vi "MW区收.vi"(6 "数值类型":enum16{"长整型", "双精度"}(ring), 7 "MD模式":enum16{"读MD", "写MD"}(ring), 9 "16#字符串":string, 10 "寄存器MD地址":i32=10, 11 "处理识别码":i32) -> (1 "数值":sgl, 2 "数值":u32, 3 "读写OK":bool)   [LabVIEW 2016]
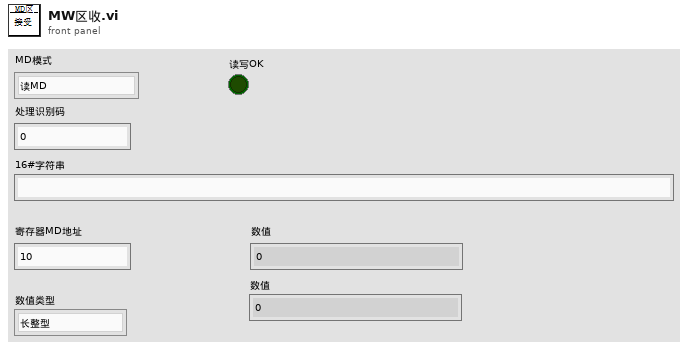
[diagram p1: front panel]
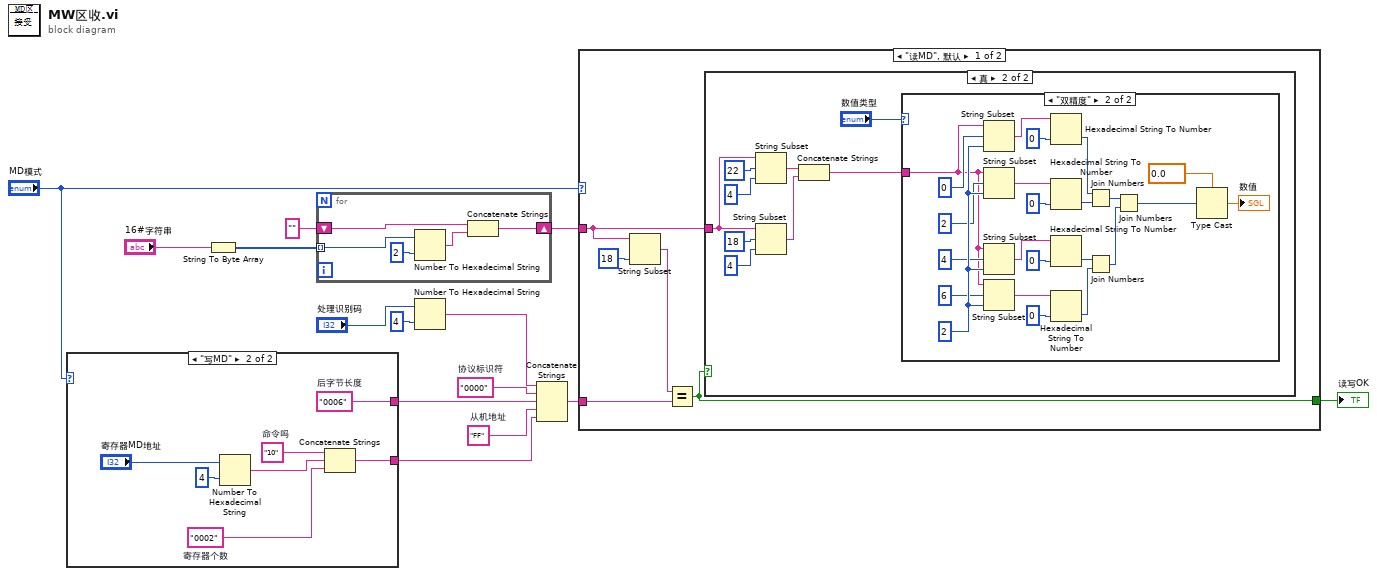
[diagram p0: block diagram]
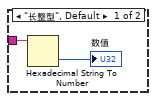
[diagram p3: hidden frame]
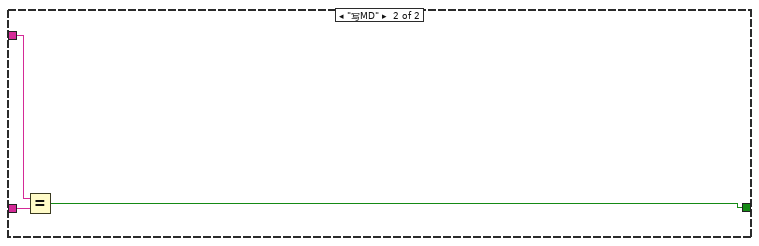
[diagram p4: hidden frame]
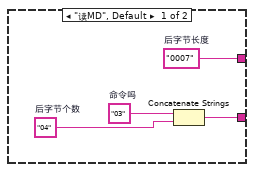
[diagram p5: hidden frame]
diagram:
  w10 = "FF"  # 从机地址
  w11 = "0000"  # 协议标识符
  n1 = case shown="\"写MD\"" "MD模式" {
    tunnel: [w18 w25] -> w9
    tunnel: [w15 w20] -> w4
    frame "读MD", Default {
      w17 = "03"  # 命令吗
      w16 = "04"  # 后字节个数
      w18 = "0007"  # 后字节长度
      n2 = Concatenate Strings(w17, w16) -> (w15:string)
    }
    frame "写MD" {
      w23 = "10"  # 命令吗
      w21 = "0002"  # 寄存器个数
      w25 = "0006"  # 后字节长度
      n3 = Number To Hexadecimal String(1:i16 4 ("宽度(-)"), 2:"寄存器MD地址") -> (0:w22:string)
      n4 = Concatenate Strings(w23, w22, w21) -> (w20:string)
    }
  }
  n5 = String To Byte Array(string="16#字符串") -> (unsigned byte array=w8:u8[])
  n6 = for {
    tunnel: w8 -> [w30] mode=indexing
    shift-right: [w28] -> w5
    shift-left: "" -> [w29]
    n7 = Number To Hexadecimal String ("数值至十六进制字符串转换")(1:i16 2 ("宽度(-)"), 2:w30) -> (0:w26:string)
    n8 = Concatenate Strings(w29, w26) -> (w28:string)
  }
  n9 = Number To Hexadecimal String(1:i16 4 ("宽度(-)"), 2:"处理识别码") -> (0:w12:string)
  n10 = Concatenate Strings(w12, w11, w9, w10, w4) -> (w2:string)
  n11 = case shown="\"读MD\", 默认" "MD模式" {
    tunnel: w5 -> [w31 w72]
    tunnel: w2 -> [w33 w71]
    tunnel: [w32 w70] -> w1
    frame "读MD", Default {
      n12 = String Subset(string=w31, length (rest)=18 ("长度（剩余）")) -> (substring=w34:string)  [unwired: 1 in]
      n13 = Equal?(x=w34, y=w33) -> (x = y?=w32:bool)
      n14 = case shown="真" w32 {
        tunnel: w31 -> [_ w38]
        frame False {
        }
        frame True {
          n15 = String Subset(string=w38, offset (0)=22 ("偏移量(0)"), length (rest)=4 ("长度（剩余）")) -> (substring=w40:string)
          n16 = String Subset(string=w38, offset (0)=18 ("偏移量(0)"), length (rest)=4 ("长度（剩余）")) -> (substring=w39:string)
          n17 = Concatenate Strings(w40, w39) -> (w36:string)
          n18 = case shown="\"双精度\"" "数值类型" {
            tunnel: w36 -> [w45 w47]
            frame "长整型", Default {
              n19 = Hexadecimal String To Number(string=w45) -> (number=→"数值":u32)  [unwired: 2 in, 1 out]
            }
            frame "双精度" {
              w52 = 2 ("长度（剩余）")
              n20 = String Subset(string=w47, offset (0)=0 ("偏移量(0)"), length (rest)=w52) -> (substring=w56:string)
              n21 = String Subset(string=w47, offset (0)=2 ("长度（剩余）"), length (rest)=w52) -> (substring=w55:string)
              n22 = String Subset(string=w47, offset (0)=4 ("长度（剩余）"), length (rest)=w52) -> (substring=w54:string)
              n23 = String Subset(string=w47, offset (0)=6 ("长度（剩余）"), length (rest)=w52) -> (substring=w53:string)
              n24 = Hexadecimal String To Number(string=w56, default (0uL)=i8 0 ("默认(0 U32)")) -> (number=w61:i8)  [unwired: 1 in, 1 out]
              n25 = Hexadecimal String To Number(string=w55, default (0uL)=i8 0 ("默认(0 U32)")) -> (number=w62:i8)  [unwired: 1 in, 1 out]
              n26 = Hexadecimal String To Number(string=w54, default (0uL)=i8 0 ("默认(0 U32)")) -> (number=w63:i8)  [unwired: 1 in, 1 out]
              n27 = Hexadecimal String To Number(string=w53, default (0uL)=i8 0 ("默认(0 U32)")) -> (number=w64:i8)  [unwired: 1 in, 1 out]
              n28 = Join Numbers(hi=w61, lo=w62) -> ((hi.lo)=w65:u16)
              n29 = Join Numbers(hi=w63, lo=w64) -> ((hi.lo)=w66:u16)
              n30 = Join Numbers(hi=w65, lo=w66) -> ((hi.lo)=w67:u32)
              n31 = Type Cast(type=sgl 0.0, x=w67) -> (*(type *) &x=→"数值":sgl)
            }
          }
        }
      }
    }
    frame "写MD" {
      n32 = Equal?(x=w72, y=w71) -> (x = y?=w70:bool)
    }
  }
  "读写OK" <- w1
